vi "Write ALR_ON_OFF_modified.vi"(8 "error in (no error)":errorcluster, 10 "modified (0)":u16, 11 "ALR in":T1) -> (0 "error out":errorcluster, 3 "ALR out":T1)   [LabVIEW 2019, in "Alarms.lvlib"]
uses:
  Alarms.lvlib
  Ctl/Alarms.ctl
  Ctl/ALR_defs.ctl
  Ctl/ALRs_State.ctl
  Ctl/ALR_ON_OFF.ctl
  Ctl/ALR_Parameters.ctl
  Ctl/ALR code.ctl
  Ctl/ALR type.ctl
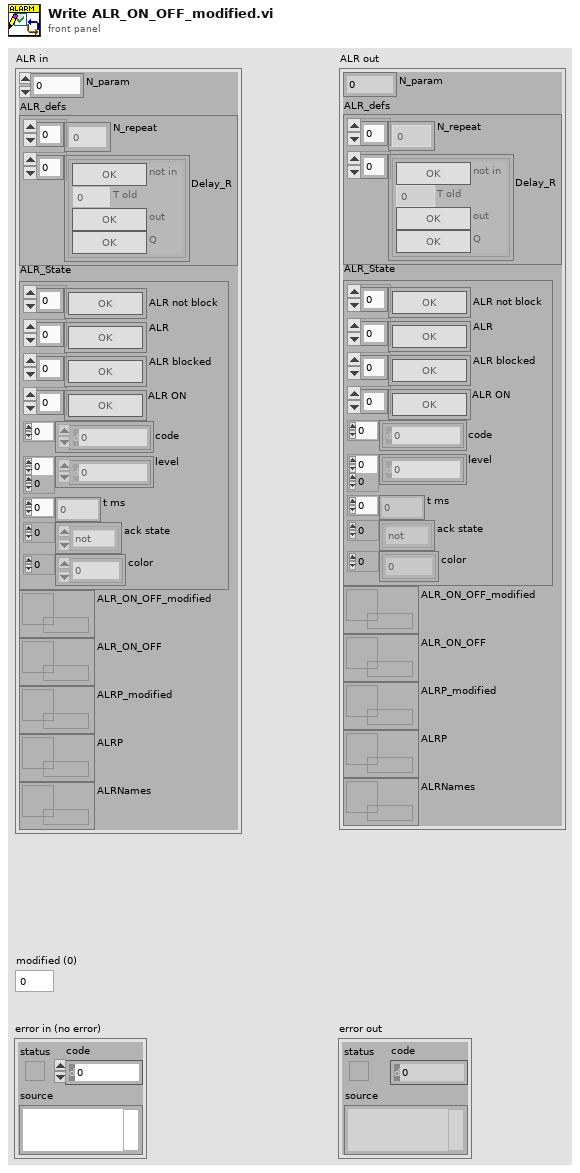
[diagram p1: front panel]
types:
  T1 = typedef "Alarms.lvlib/Alarms.ctl" = cluster{"N_param":i32, "ALR_defs":T2, "ALR_State":T3, "ALR_ON_OFF_modified":refnum<data-value>, "ALR_ON_OFF":refnum<data-value>, "ALRP_modified":refnum<data-value>, "ALRP":refnum<data-value>, "ALRNames":refnum<data-value>}
  T2 = typedef "Alarms.lvlib/ALR_defs.ctl" = cluster{"N_repeat":u32[], "Delay_R":cluster{"not in":bool, "T old":u32, "out":bool, "Q":bool}[]}
  T3 = typedef "Alarms.lvlib/ALRs_State.ctl" = cluster{"ALR not block":bool[], "ALR":bool[], "ALR blocked":bool[], "ALR ON":bool[], "code":i32[], "level":i32[][], "t ms":u32[], "ack state":enum32{"not", "tripped", "reset", "ack"}[], "color":u32[]}
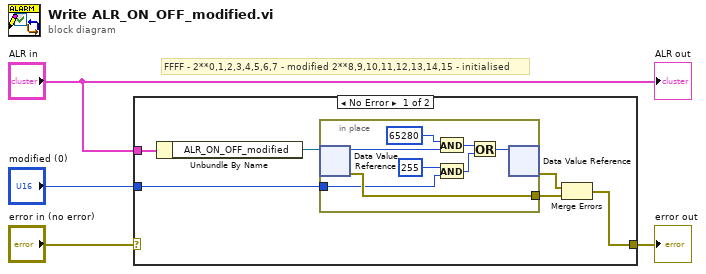
[diagram p0: block diagram]
diagram:
  # "FFFF - 2**0,1,2,3,4,5,6,7 - modified 2**8,9,10,11,12,13,14,15 - initialised"
  n1 = case shown="No Error" "error in (no error)" {
    selector: "error in (no error)" -> [_ w19]
    tunnel: [w10 w19] -> w3
    tunnel: "ALR in" -> [w9 _]
    tunnel: "modified (0)" -> [w7 _]
    frame No Error {
      n2 = Unbundle By Name(w9) -> ("ALR_ON_OFF_modified"=w8:refnum<data-value>)
      n3 = in-place {
        in-place-border: w7 -> [w15]
        in-place-border: [w18] -> w6
        n4 = in-place-dvr #1(w8) -> (w16:u16, w18:errorcluster)
        n5 = And(x=u16 65280, y=w16) -> (x .and. y?=w17:u16)
        n6 = And(x=u16 255, y=w15) -> (x .and. y?=w14:u16)
        n7 = Or(x=w17, y=w14) -> (x .or. y?=w13:u16)
        n8 = in-place-dvr #1(w13) -> (w5:errorcluster)  [unwired: 1 out]
      }
      n9 = Merge Errors(w5, w6) -> (w10:errorcluster)
    }
    frame Error {
    }
  }
  "error out" <- w3
  "ALR out" <- "ALR in"
